vi "Send Process Calculation Results.vi"(7 "Message Priority (Normal)":T2=enum."Normal", 8 "error in (no error)":errorcluster, 10 "Calculation Results":T1, 11 "Message Enqueuer":refnum<class "Message Enqueuer.lvclass">) -> (0 "error out":errorcluster, 3 "Message Enqueuer out":refnum<class "Message Enqueuer.lvclass">)   [LabVIEW 2020, in "CPU FFT Calculator.lvlib" / "Process Calculation Results Msg.lvclass"]
doc: "This VI sends the message to an actor."
uses:
  Process Calculation Results Msg.lvclass
  <vilib>/ActorFramework/Message Enqueuer/Message Enqueuer.lvclass
  <vilib>/ActorFramework/Message Enqueuer/Message Priority.ctl
  CPU FFT Calculator/CPU Calculation Results.ctl
  C:/Program Files/National Instruments/LabVIEW 2026/vi.lib/ActorFramework/Message/Message.lvclass
  Process Calculation Results Msg.lvclass/Process Calculation Results Msg.ctl
  <vilib>/ActorFramework/Message Enqueuer/Message Enqueuer.lvclass/Message Enqueuer.ctl
  <vilib>/ActorFramework/Message Priority Queue/Priority Enqueue.vi
  CPU FFT Calculator/CPU FFT Calculator.lvclass
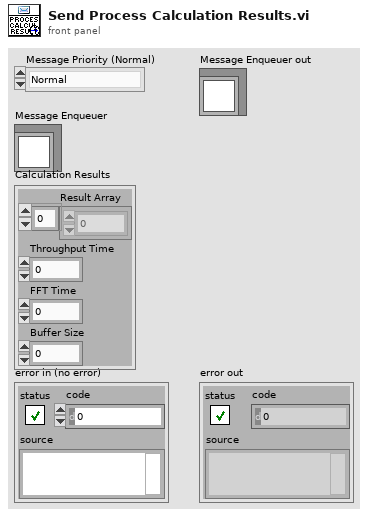
[diagram p1: front panel]
types:
  T1 = typedef "CPU FFT Calculator.lvlib/CPU FFT Calculator.lvclass/CPU Calculation Results.ctl" = cluster{"Result Array":sgl[], "Throughput Time":dbl, "FFT Time":dbl, "Buffer Size":i32}
  T2 = typedef "Actor Framework.lvlib/Message Enqueuer.lvclass/Message Priority.ctl" = enum16{"Low", "Normal", "High"}
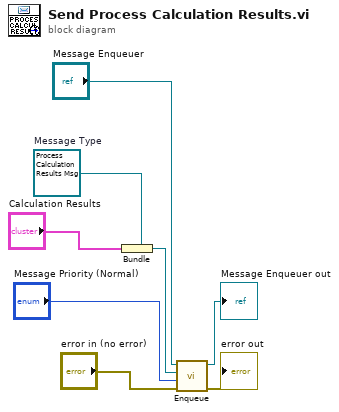
[diagram p0: block diagram]
diagram:
  w2 = refnum<class "Process Calculation Results Msg.lvclass"> refnum  # Message Type
  n1 = Bundle(cluster=w2, "Calculation Results") -> (w3:refnum<class "Process Calculation Results Msg.lvclass">)
  n2 = call <vilib>:"Enqueue.vi"("error in (no error)"="error in (no error)", "Message Priority (Normal)"="Message Priority (Normal)", "Message"=w3, "Message Enqueuer in"="Message Enqueuer") -> ("error out"=→"error out":errorcluster, "Message Enqueuer out"=→"Message Enqueuer out":refnum<class "Message Enqueuer.lvclass">)  [unwired: 6 in]
